vi "PIDController_GetContinuousError.vi"(10 "Error":dbl, 11 "in PID_CONTROLLER":T1={"Kp"=0.0, "Ki"=0.0, "Kd"=0.0, "Period"=0.0, "Max_Integral"=0.0, "Min_Integral"=0.0, "Max_Input"=0.0, "Min_Input"=0.0, "Input_Range"=0.0, "Continuous"=FALSE, "PositionError"=0.0, "VelocityError"=0.0, "PrevError"=0.0, "TotalError"=0.0, "PositionTolerance"=0.0, "VelocityTolerance"=0.0, "SetPoint"=0.0, "Kf"=0.0, "Prev_Deriv"=0.0, "Prev_Deriv 2"=0.0, "DerivativeFilter"=FALSE, "Min_Output"=-9.99e+35, "Max_Output"=9.9e+35, "Prev_F_P"=0.0, "Prev_F_P_2"=0.0, "AntiWindupActive"=FALSE} {"Prev_F_P_2" format="%16_6e"; "Prev_F_P" format="%16_6e"; "Max_Output" format="%16_6e"; "Min_Output" format="%16_6e"; "Prev_Deriv 2" format="%17.6f"; "Prev_Deriv" format="%17.6f"; "Kf" format="%17.6f"; "SetPoint" format="%17.6f"; "VelocityTolerance" format="%17.6f"; "PositionTolerance" format="%17.6f"; "TotalError" format="%17.6f"; "PrevError" format="%17.6f"; "VelocityError" format="%17.6f"; "PositionError" format="%17.6f"; "Input_Range" format="%17.6f"; "Min_Input" format="%17.6f"; "Max_Input" format="%17.6f"; "Min_Integral" format="%17.6f"; "Max_Integral" format="%17.6f"; "Period" format="%17.6f"; "Kd" format="%17.6f"; "Ki" format="%17.6f"; "Kp" format="%17.6f"}) -> (3 "ContinousError":dbl)   [LabVIEW 2019, in "Trajectory_Library.lvlib"]
doc: "Wraps error around for continuous inputs. The original error is returned if continuous mode is disabled.\n \nInputs:\n - PID_Controller -- PID_Controller data cluster\n - error -- The current error of the PID controller.\n\nOutputs:\n - ContinuousError -- Error for continuous inputs."
uses:
  Trajectory_Library.lvlib
  PID_CONTROLLER.ctl
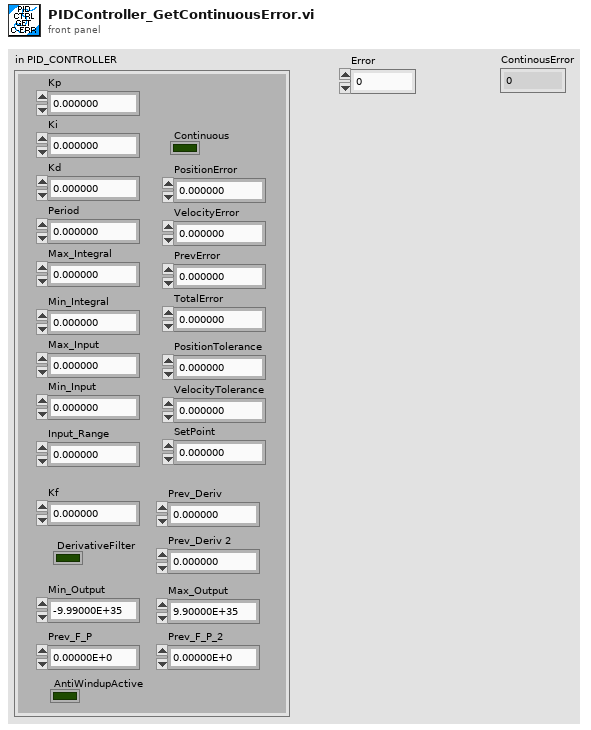
[diagram p1: front panel]
types:
  T1 = typedef "Trajectory_Library.lvlib/PID_CONTROLLER.ctl" = cluster{"Kp":dbl, "Ki":dbl, "Kd":dbl, "Period":dbl, "Max_Integral":dbl, "Min_Integral":dbl, "Max_Input":dbl, "Min_Input":dbl, "Input_Range":dbl, "Continuous":bool, "PositionError":dbl, "VelocityError":dbl, "PrevError":dbl, "TotalError":dbl, "PositionTolerance":dbl, "VelocityTolerance":dbl, "SetPoint":dbl, "Kf":dbl, "Prev_Deriv":dbl, "Prev_Deriv 2":dbl, "DerivativeFilter":bool, "Min_Output":dbl, "Max_Output":dbl, "Prev_F_P":dbl, "Prev_F_P_2":dbl, "AntiWindupActive":bool}
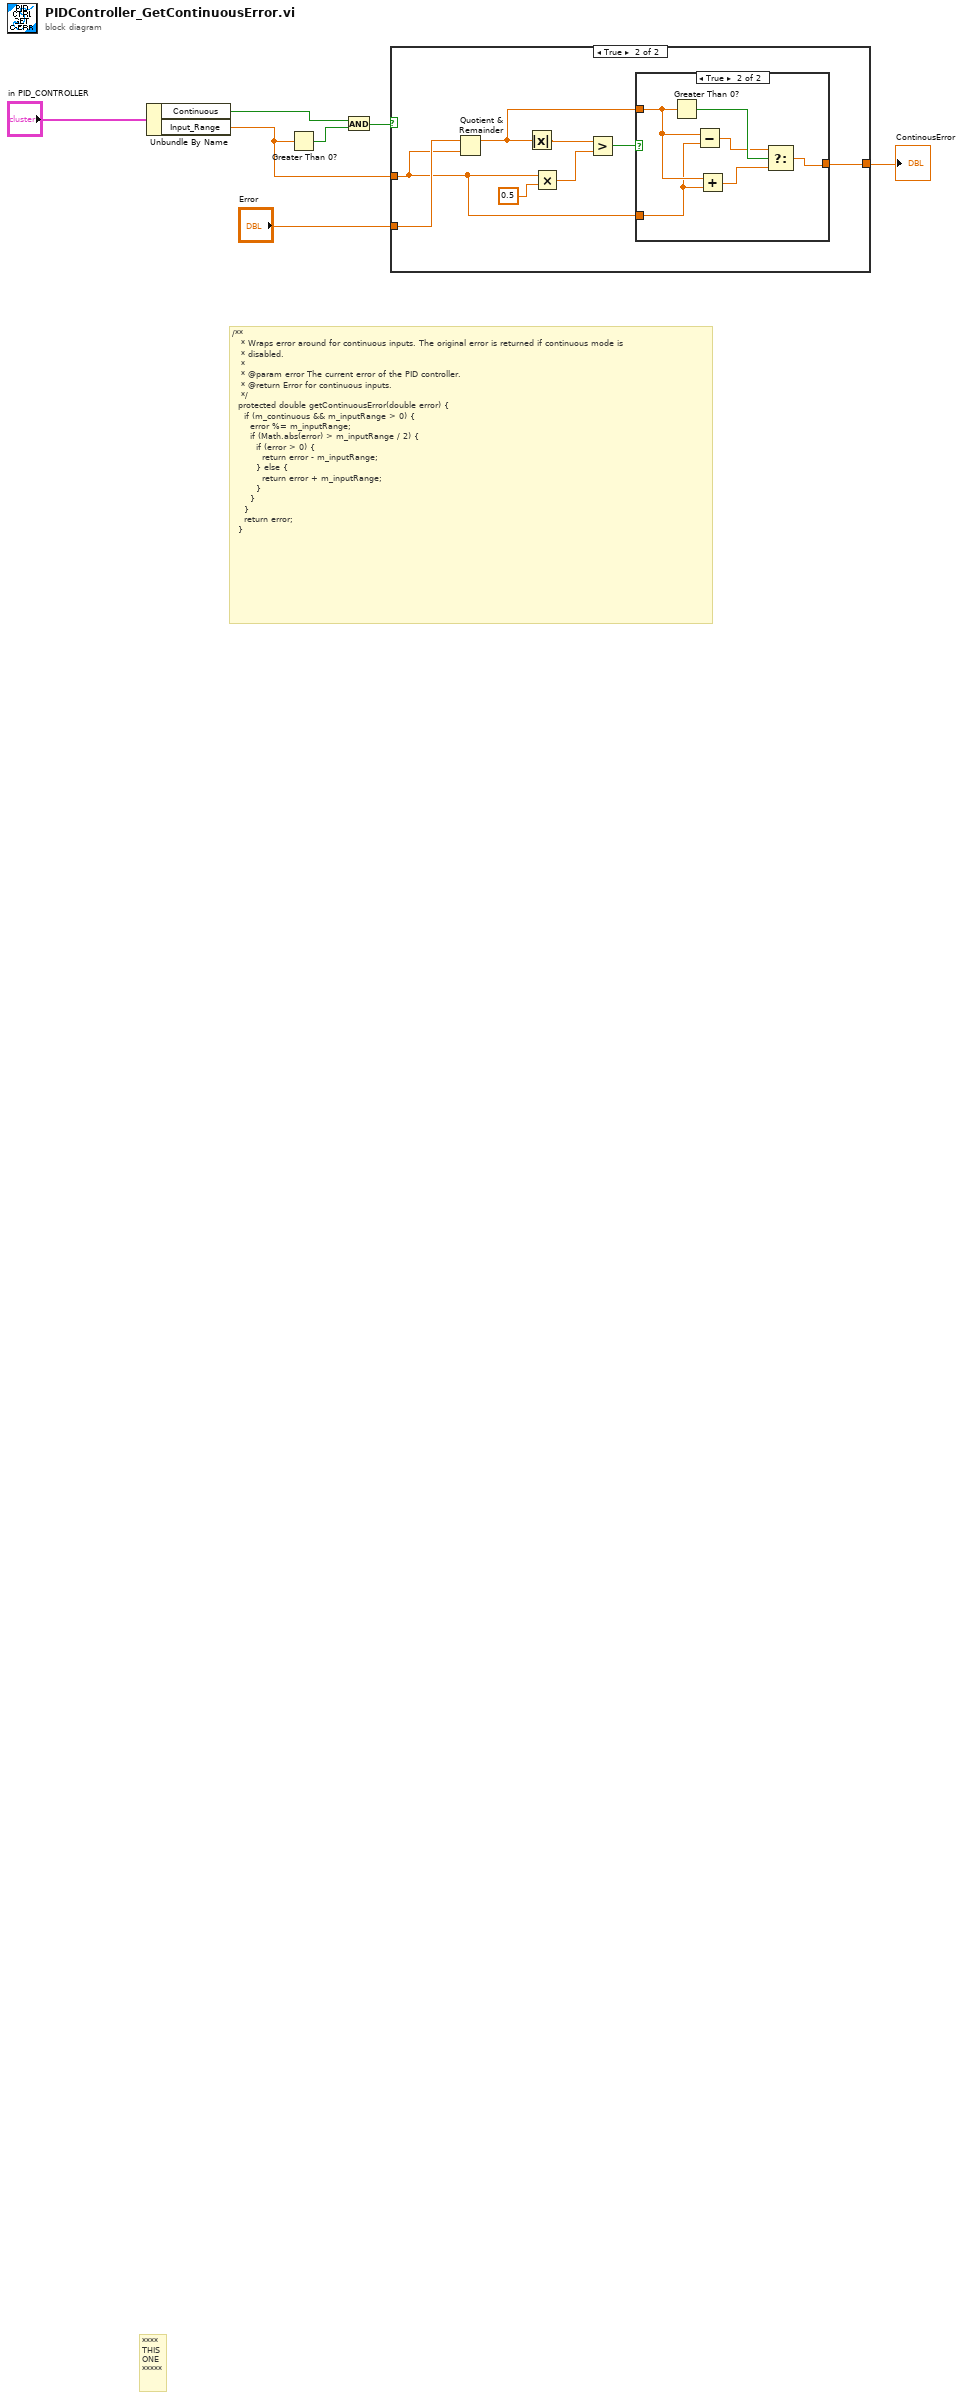
[diagram p0: block diagram]
diagram:
  # "/**\n   * Wraps error around for continuous inputs. The original error is returned if continuous mode is\n   * disabled.\n   *\n   * @param error The current error of the PID controller.\n   * @return Error for continuous inputs.\n   */\n  protected double getContinuousError(double error) {\n    if (m_continuous && m_inputRange > 0) {\n      error %= m_inputRange;\n      if (Math.abs(error) > m_inputRange / 2) {\n        if (error > 0) {\n          return error - m_inputRange;\n        } else {\n          return error + m_inputRange;\n        }\n      }\n    }\n    return error;\n  }"
  # "****\nTHIS\nONE\n*****"
  n1 = Unbundle By Name("in PID_CONTROLLER") -> ("Continuous"=w6:bool, "Input_Range"=w1:dbl)
  n2 = Greater Than 0?(x=w1) -> (x > 0?=w5:bool)
  n3 = And(x=w6, y=w5) -> (x .and. y?=w4:bool)
  n4 = case shown="True" w4 {
    tunnel: "Error" -> [w8 w16]
    tunnel: [w8 w11] -> w2
    tunnel: w1 -> [_ w9]
    frame False {
    }
    frame True {
      n5 = Quotient & Remainder(x=w16, y=w9) -> (x-y*floor(x/y)=w10:dbl)  [unwired: 1 out]
      n6 = Absolute Value(x=w10) -> (abs(x)=w14:dbl)
      n7 = Multiply(x=w9, y=0.5) -> (x*y=w13:dbl)
      n8 = Greater?(x=w14, y=w13) -> (0:w12:bool)
      n9 = case shown="True" w12 {
        tunnel: [w17 w18] -> w11
        tunnel: w10 -> [w17 w22]
        tunnel: w9 -> [_ w21]
        frame False {
        }
        frame True {
          n10 = Greater Than 0?(x=w22) -> (x > 0?=w23:bool)
          n11 = Subtract(x=w22, y=w21) -> (x-y=w20:dbl)
          n12 = Add(x=w22, y=w21) -> (x+y=w19:dbl)
          n13 = Select(t=w20, s=w23, f=w19) -> (s? t:f=w18:dbl)
        }
      }
    }
  }
  "ContinousError" <- w2
